vi "tempConvert.vi"(9 "Units":string, 11 "ticks":dbl) -> (3 "value":dbl)   [LabVIEW 2012]
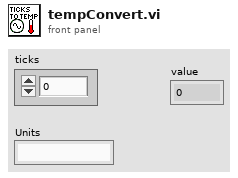
[diagram p1: front panel]
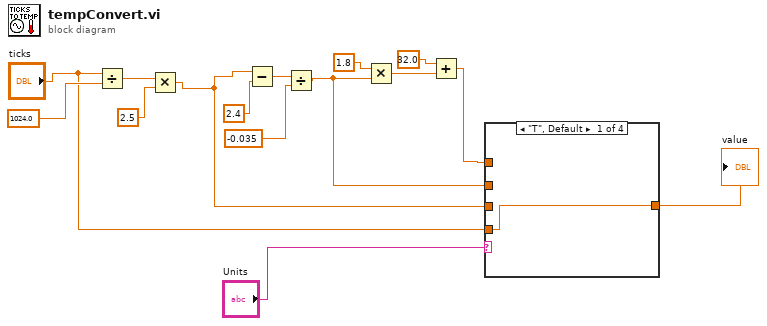
[diagram p0: block diagram]
diagram:
  n1 = Divide(x="ticks", y=1024.0) -> (x/y=w14:dbl)
  n2 = Multiply(x=w14, y=2.5) -> (x*y=w6:dbl)
  n3 = Subtract(x=w6, y=2.4 ("x")) -> (x-y=w4:dbl)
  n4 = Divide(x=w4, y=-0.035 ("x")) -> (x/y=w3:dbl)
  n5 = Multiply(x=1.8, y=w3) -> (x*y=w12:dbl)
  n6 = Add(x=32.0, y=w12) -> (x+y=w7:dbl)
  n7 = case shown="\"T\", Default" "Units" {
    tunnel: [w16 w17 w18 w19] -> w8
    tunnel: w6 -> [_ _ _ w19]
    tunnel: w3 -> [_ _ w18 _]
    tunnel: w7 -> [_ w17 _ _]
    tunnel: "ticks" -> [w16 _ _ _]
    frame "T", Default {
    }
    frame "F" {
    }
    frame "C" {
    }
    frame "V" {
    }
  }
  "value" <- w8
